vi "Initialize Logging.vi"(8 "error in":errorcluster, 10 "Custom Device Name":string, 11 "Custom Device in":refnum<class "NIDMM Engine.lvclass">) -> (0 "error out":errorcluster, 3 "Custom Device out":refnum<class "NIDMM Engine.lvclass">)   [LabVIEW 2026, in "NIDMM Engine.lvlib" / "NIDMM Engine.lvclass"]
uses:
  NIDMM Engine.lvclass
  NIDMM Engine.lvclass/NIDMM Engine.ctl
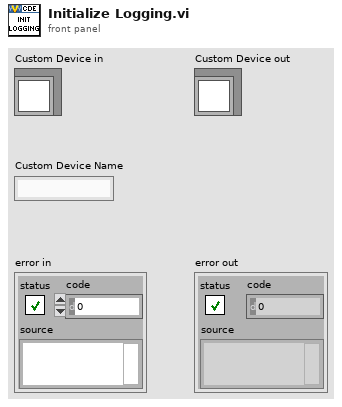
[diagram p1: front panel]
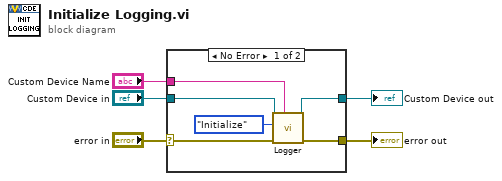
[diagram p0: block diagram]
diagram:
  n1 = case shown="No Error" "error in" {
    selector: "error in" -> [w11 w13]
    tunnel: [w10 w13] -> w4
    tunnel: [w8 w12] -> w2
    tunnel: "Custom Device in" -> [w9 w12]
    tunnel: "Custom Device Name" -> [w7 _]
    frame No Error {
      n2 = call "Logger.vi"("Custom Device Name"=w7, "error in"=w11, "State"=enum16{"Initialize", "Log"}."Initialize", "Custom Device in"=w9) -> ("error out"=w10:errorcluster, "Custom Device out"=w8:refnum<class "NIDMM Engine.lvclass">)  [unwired: 6 in]
    }
    frame Error {
    }
  }
  "error out" <- w4
  "Custom Device out" <- w2
